vi "Merge Error.vi"(10 "Error":errorcluster, 11 "Set Error in":refnum<class "jettl Event Actor.lvclass">) -> (3 "Set Error out":refnum<class "jettl Event Actor.lvclass">)   [LabVIEW 2021, in "jettl Event Actor.lvlib" / "jettl Event Actor.lvclass"]
uses:
  jettl Event Actor.lvclass
  jettl Event Actor.lvclass/jettl Event Actor.ctl
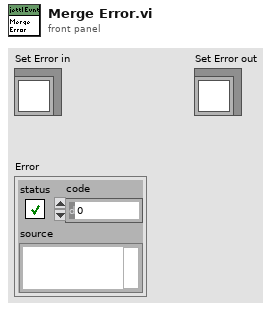
[diagram p1: front panel]
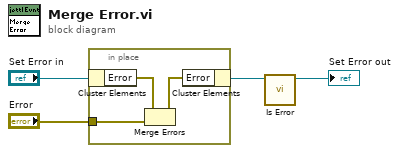
[diagram p0: block diagram]
diagram:
  n1 = in-place {
    in-place-border: "Error" -> [w5]
    n2 = in-place-cluster #1("Set Error in") -> ("Error"=w7:errorcluster)
    n3 = Merge Errors(w7, w5) -> (w6:errorcluster)
    n4 = in-place-cluster #1("Error"=w6) -> (w2:refnum<class "jettl Event Actor.lvclass">)
  }
  n5 = call "Is Error.vi"("jettl Event Actor in"=w2) -> ("jettl Event Actor out"=→"Set Error out":refnum<class "jettl Event Actor.lvclass">)  [unwired: 10 in]
